vi "init.vi"(8 "error in (no error)":errorcluster, 10 "side":dbl, 11 "Square in":refnum<class "Square.lvclass">) -> (0 "error out":errorcluster, 3 "Square out":refnum<class "Square.lvclass">)   [LabVIEW 2024, in "Square.lvclass"]
uses:
  Square.lvclass
  Square.lvclass/Square.ctl
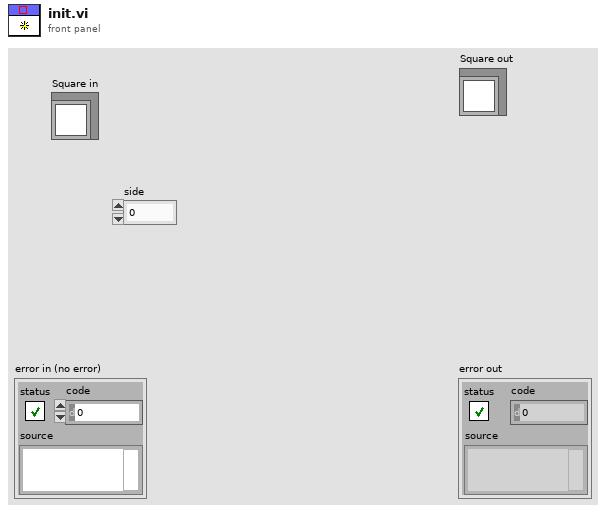
[diagram p1: front panel]
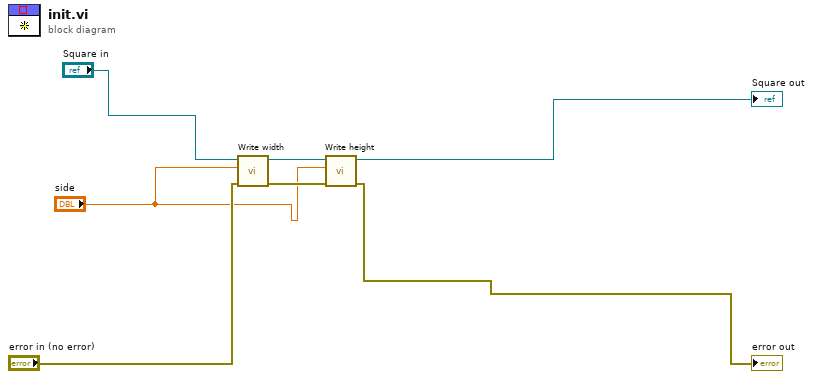
[diagram p0: block diagram]
diagram:
  n1 = call-dynamic "Write width.vi"("error in (no error)"="error in (no error)", "width"="side", "Rectangle in"="Square in") -> ("error out"=w7:errorcluster, "Rectangle out"=w5:refnum<class "Square.lvclass">)  [unwired: 7 in]
  n2 = call-dynamic "Write height.vi"("error in (no error)"=w7, "height"="side", "Rectangle in"=w5) -> ("error out"=→"error out":errorcluster, "Rectangle out"=→"Square out":refnum<class "Square.lvclass">)  [unwired: 7 in]
